vi "Pressure_transducer_practice.vi"() -> ()   [LabVIEW 2014]
panel:
  out "Data array":dbl[](array[numeric])
  out "Darta from Transducer":dynamicdata(graph) caption="data"
  in  "stop (F)":bool
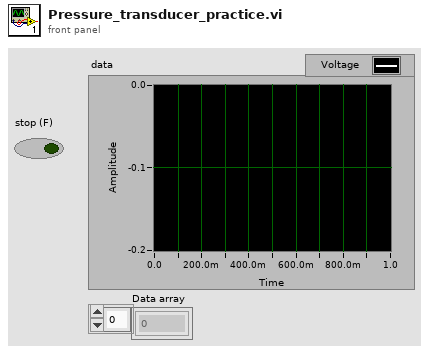
[diagram p1: front panel]
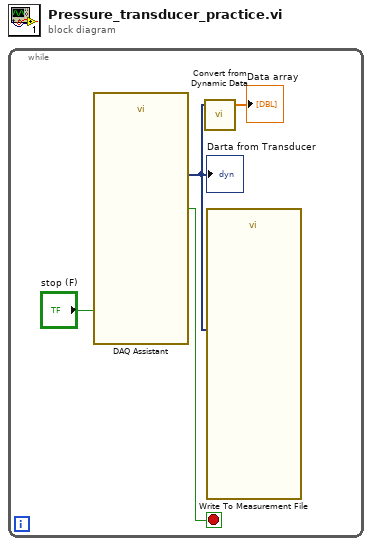
[diagram p0: block diagram]
diagram:
  n1 = while {
    stop <- w3 stop-if-true
    n2 = call "DAQ Assistant"("stop (F)"="stop (F)") -> ("data"=w1:dynamicdata, "stopped"=w3:bool)  [unwired: 15 in, 2 out]
    "Darta from Transducer" <- w1
    n3 = call "Convert from Dynamic Data"("Dynamic Data Type"=w1) -> ("Array"=→"Data array":dbl[])  [unwired: 3 in]
    n4 = call "Write To Measurement File"("Signals"=w1) -> ()  [unwired: 16 in, 3 out]
  }
